vi "Pad Message.vi"(11 "Message Byte Array":u8[](array[numeric])) -> (3 "Padded Message":u32[](array[numeric]), 5 "Chunks":i32)   [LabVIEW 2018, in "Crypto.lvlib" / "SHA-256.lvclass"]
uses:
  SHA-256.lvclass
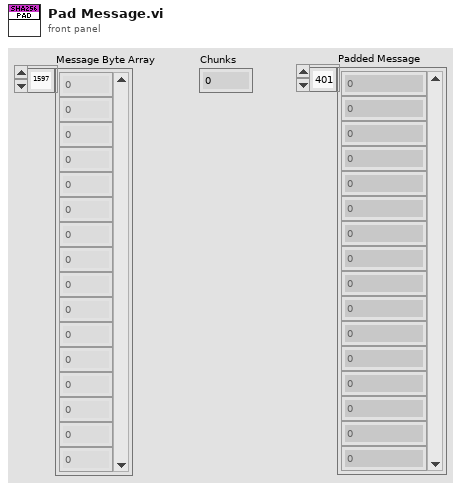
[diagram p1: front panel]
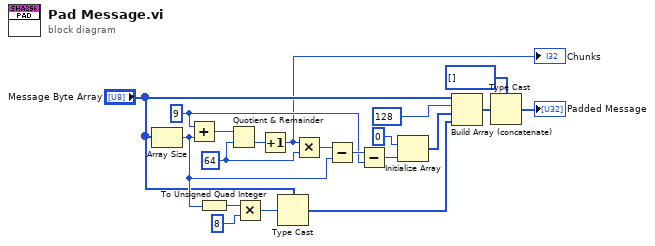
[diagram p0: block diagram]
diagram:
  w14 = 64 ("y")
  w7 = 9 ("x")
  n1 = Array Size(array="Message Byte Array") -> (size(s)=w16:i32)
  n2 = Add(x=w7, y=w16) -> (x+y=w12:i32)
  n3 = To Unsigned Quad Integer(1:w16) -> (0:w9:u64)
  n4 = Quotient & Remainder(x=w12, y=w14) -> (floor(x/y)=w13:i32)  [unwired: 1 out]
  n5 = Multiply(x=w9, y=u64 8 ("x")) -> (x*y=w6:u64)
  n6 = Increment(x=w13) -> (x+1=w1:i32)
  "Chunks" <- w1
  n7 = Type Cast(type="Message Byte Array", x=w6) -> (*(type *) &x=w11:u8[])
  n8 = Multiply(x=w1, y=w14) -> (x*y=w15:i32)
  n9 = Subtract(x=w15, y=w16) -> (x-y=w17:i32)
  n10 = Subtract(x=w17, y=w7) -> (x-y=w18:i32)
  n11 = Initialize Array(u8 0 ("element"), w18) -> (w20:u8[])
  n12 = Build Array (concatenate)("Message Byte Array", u8 128, w20, w11) -> (w4:u8[])
  n13 = Type Cast(type=u32[] [], x=w4) -> (*(type *) &x=→"Padded Message":u32[])
